vi "Advance past String.vi"(7 "JSON":string, 9 "Offset":i32, 11 "State in":T1=enum."String") -> (1 "Offset past match":i32, 3 "State":T1, 6 "Value start out":i32)   [LabVIEW 2017, in "JSONtext.lvlib"]
uses:
  JSONtext.lvlib
  Parsing State.ctl
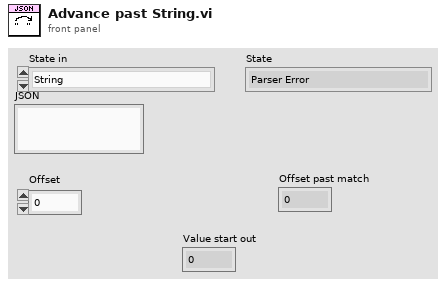
[diagram p1: front panel]
types:
  T1 = typedef "JSONtext.lvlib/Parsing State.ctl" = enum16{"Parser Error", "Object", "Array", "String", "Number/Other", "Leading Whitespace", "Object end", "Array end", "Value end"}
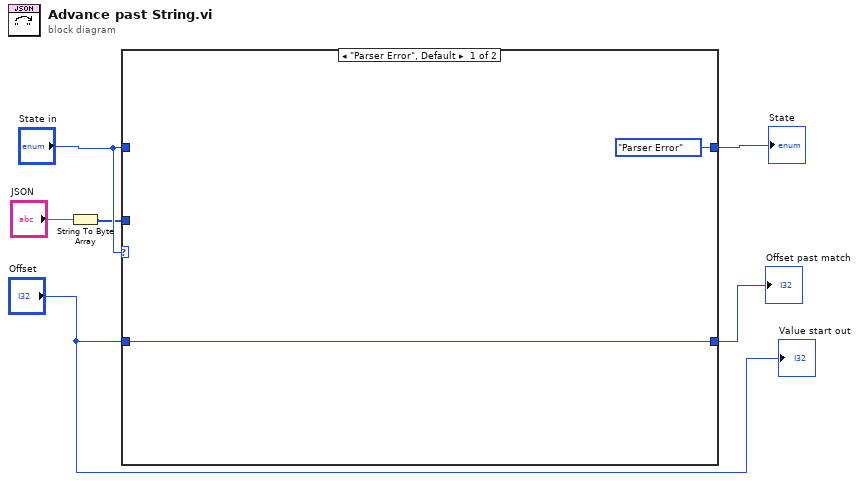
[diagram p0: block diagram]
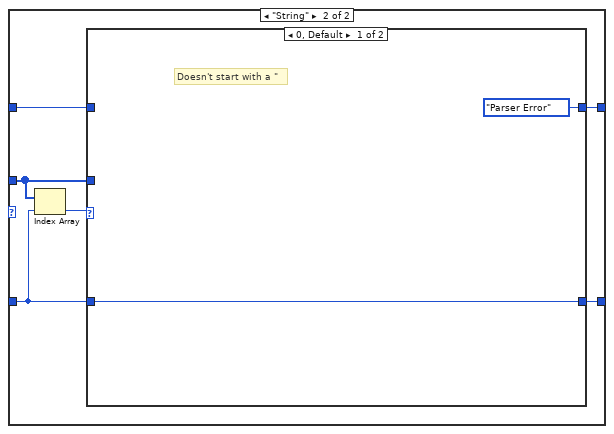
[diagram p2: hidden frame]
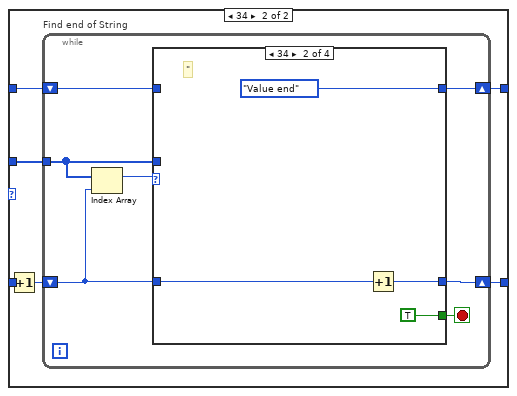
[diagram p3: hidden frame]
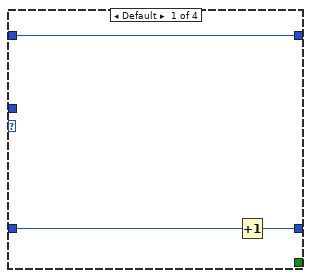
[diagram p4: hidden frame]
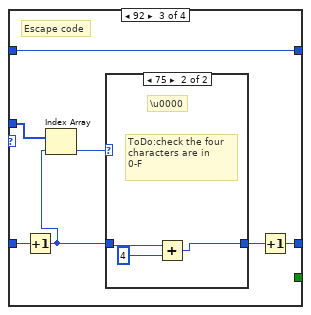
[diagram p5: hidden frame]
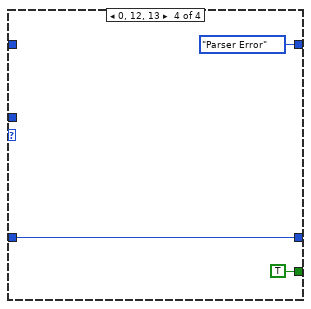
[diagram p7: hidden frame]
diagram:
  n1 = String To Byte Array(string="JSON") -> (unsigned byte array=w1:u8[])
  n2 = case shown="\"Parser Error\", Default" "State in" {
    tunnel: [Parsing_State."Parser Error" ("State in") w14] -> w6
    tunnel: [w8 w13] -> w5
    tunnel: w1 -> [_ w11]
    tunnel: "State in" -> [_ w12]
    tunnel: "Offset" -> [w8 w10]
    frame "Parser Error", Default {
    }
    frame "String" {
      n3 = Index Array(array=w11, index=w10) -> (element=w9:u8)
      n4 = case shown="0, Default" w9 {
        tunnel: [Parsing_State."Parser Error" ("State in") w22] -> w14
        tunnel: [w15 w21] -> w13
        tunnel: w12 -> [_ w20]
        tunnel: w11 -> [_ w18]
        tunnel: w10 -> [w15 w17]
        frame 0, Default {
          # "Doesn't start with a \""
        }
        frame 34 {
          n5 = Increment(x=w17) -> (x+1=w19:i32)
          n6 = while "Find end of String" {
            tunnel: w18 -> [w28]
            shift-right: [w23] -> w21
            shift-left: w19 -> [w24]
            shift-right: [w26] -> w22
            shift-left: w20 -> [w27]
            stop <- w25 stop-if-true
            n7 = Index Array(array=w28, index=w24) -> (element=w29:u8)
            n8 = case shown="34" w29 {
              tunnel: w28 -> [_ _ w41 _]
              tunnel: w27 -> [w32 _ w42 _]
              tunnel: [w32 Parsing_State."Value end" w42 Parsing_State."Parser Error"] -> w26
              tunnel: [_ TRUE _ TRUE] -> w25
              tunnel: w24 -> [w31 w34 w43 w50]
              tunnel: [w30 w33 w37 w50] -> w23
              frame Default {
                n9 = Increment(x=w31) -> (x+1=w30:i32)
              }
              frame 34 {
                # "\""
                n10 = Increment(x=w34) -> (x+1=w33:i32)
              }
              frame 92 {
                # "Escape code"
                n11 = Increment(x=w43) -> (x+1=w39:i32)
                n12 = Index Array(array=w41, index=w39) -> (element=w40:u8)
                n13 = case shown="75" w40 {
                  tunnel: w39 -> [w44 w47]
                  tunnel: [w44 w45] -> w38
                  frame Default {
                    # "escaped character"
                  }
                  frame 117 {
                    # "ToDo:check the four\ncharacters are in\n0-F"
                    # "\\u0000"
                    n14 = Add(x=w47, y=4) -> (x+y=w45:i32)
                  }
                }
                n15 = Increment(x=w38) -> (x+1=w37:i32)
              }
              frame 0, 12, 13 {
              }
            }
          }
        }
      }
    }
  }
  "State" <- w6
  "Offset past match" <- w5
  "Value start out" <- "Offset"
